vi "Script Add Constant VI.vi"(4 "Project Ref":refnum<vi>, 6 "App Ref":refnum<vi>, 7 "Constant VI Name":string="TESTING.vi", 8 "error in":errorcluster, 9 "Constant VI Args":refnum<vi>, 10 "Library Reference":refnum<vi>) -> (0 "error out":errorcluster)   [LabVIEW 2020, in "ConstantErrorsMaker.lvlib"]
uses:
  ConstantErrorsMaker.lvlib
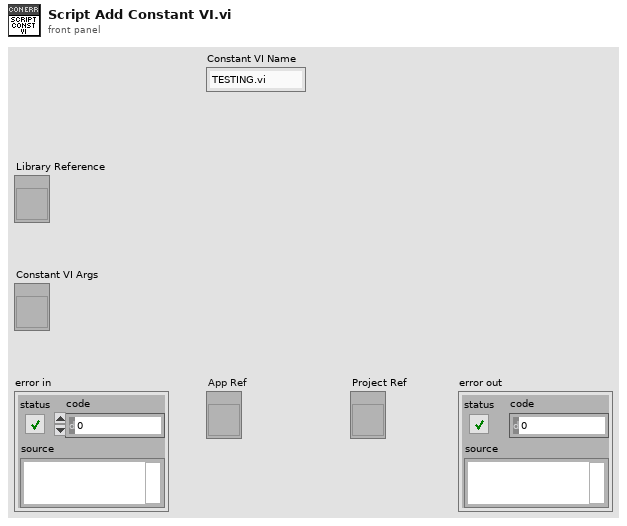
[diagram p1: front panel]
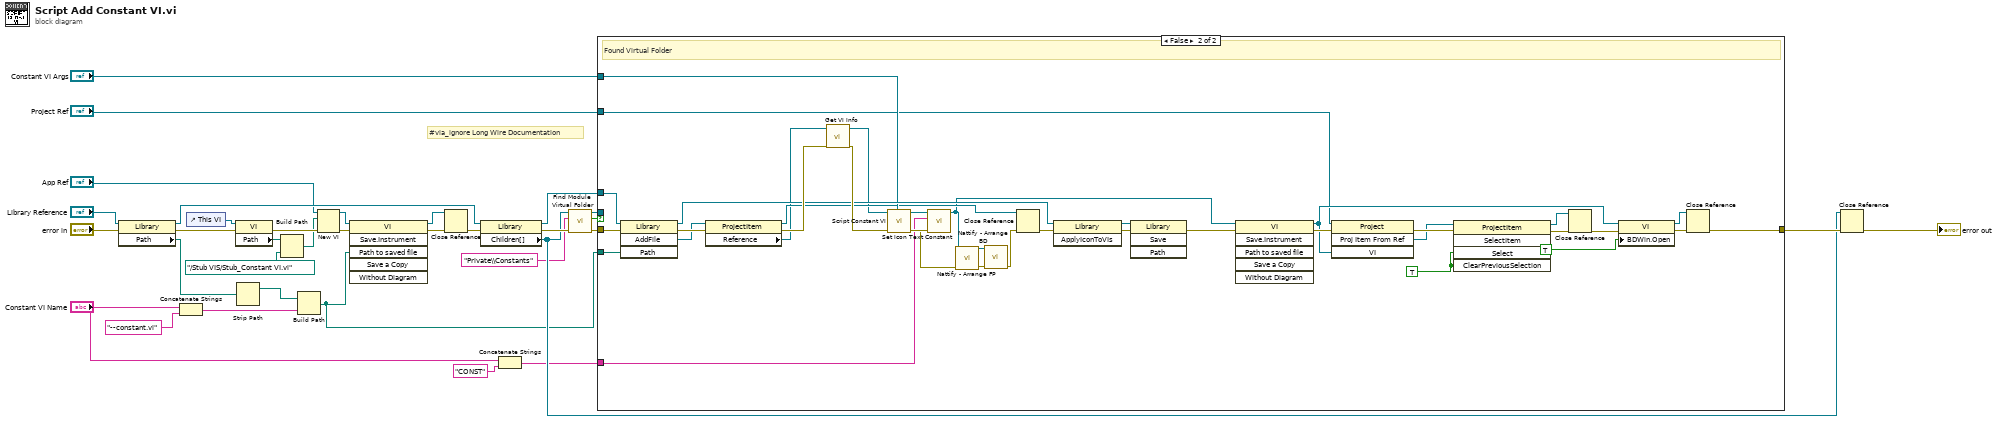
[diagram p0: block diagram]
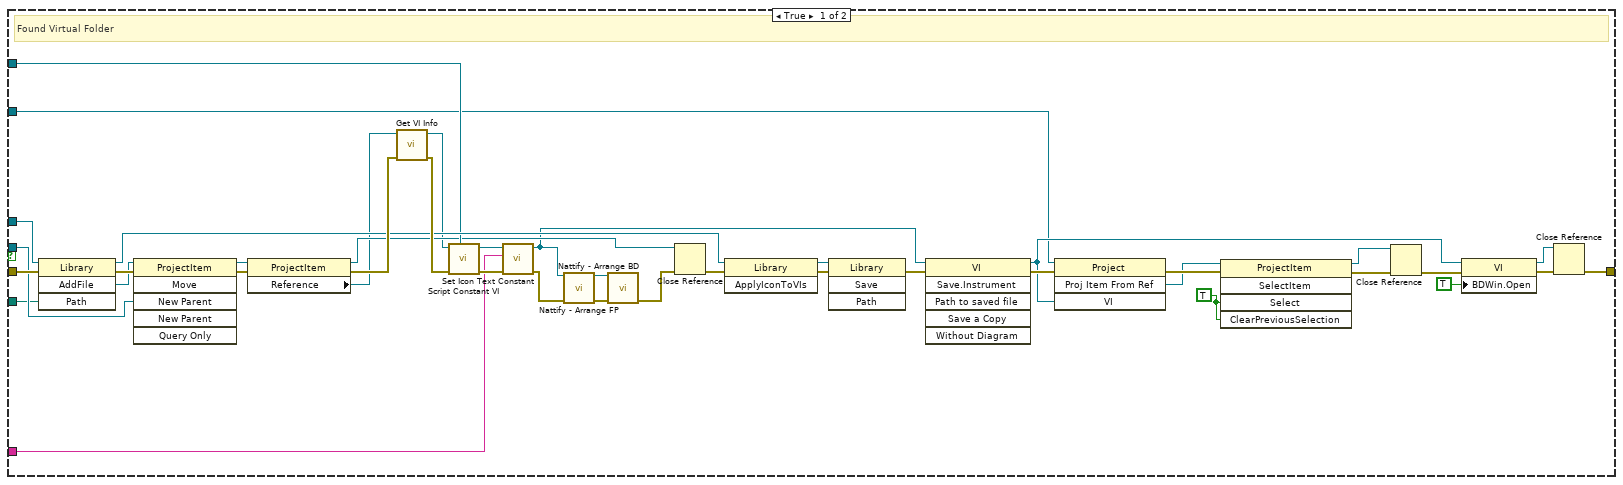
[diagram p2: hidden frame]
diagram:
  # "#via_ignore Long Wire Documentation"
  n1 = property class="Library"(reference="Library Reference", error in="error in") -> (reference out=w23:refnum<vi>, error out=w31:errorcluster, "Path"=w12:path)
  n2 = Concatenate Strings("Constant VI Name", "--constant.vi" ("input 1")) -> (w11:string)
  n3 = control-ref of="This VI"() -> (w10:refnum<vi>)
  n4 = property class="VI"(reference=w10, error in=w31) -> (error out=w25:errorcluster, "Path"=w9:path)  [unwired: 1 out]
  n5 = Strip Path(path=w12) -> (stripped path=w14:path)  [unwired: 1 out]
  n6 = Build Path(base path=w9, name or relative path=path "../Stub VIS/Stub_Constant VI.vi") -> (appended path=w8:path)
  n7 = Build Path(base path=w14, name or relative path=w11) -> (appended path=w13:path)
  n8 = New VI(8:w25, 10:w8, 11:"App Ref") -> (0:w28:errorcluster, 3:w16:refnum<vi>)  [unwired: 4 in]
  n9 = invoke class="VI" method="Save.Instrument"(reference=w16, error in=w28, "Path to saved file"=w13) -> (reference out=w6:refnum<vi>, error out=w26:errorcluster)  [unwired: 3 in, 4 out]
  n10 = Close Reference(reference=w6, error in (no error)=w26) -> (error out=w27:errorcluster)
  n11 = property class="Library"(reference=w23, error in=w27) -> (reference out=w24:refnum<vi>, error out=w33:errorcluster, "Children[]"=w20:refnum<vi>[])
  n12 = Concatenate Strings("Constant VI Name", "CONST" ("string")) -> (w2:string)
  n13 = call "Find Module Virtual Folder.vi"("error in"=w33, "Virtual Folder"="Private\\Constants", "Children"=w20) -> ("error out"=w32:errorcluster, "Found?"=w21:bool, "ProjectItem out"=w22:refnum<vi>)  [unwired: 6 in]
  n14 = case shown="False" w21 {
    tunnel: [w63 w101] -> w34
    tunnel: w24 -> [w56 w94]
    tunnel: w32 -> [w74 w111]
    tunnel: w22 -> [w54 _]
    tunnel: "Constant VI Args" -> [w50 w89]
    tunnel: w13 -> [w51 w90]
    tunnel: w2 -> [w42 w82]
    tunnel: "Project Ref" -> [w37 w78]
    frame True {
      w40 = TRUE ("Select")
      # "Found Virtual Folder"
      n15 = invoke class="Library" method="AddFile"(reference=w56, error in=w74, "Path"=w51) -> (reference out=w53:refnum<vi>, error out=w73:errorcluster, "AddFile"=w55:refnum<vi>)  [unwired: 1 in, 1 out]
      n16 = invoke class="ProjectItem" method="Move"(reference=w55, error in=w73, "New Parent"=w54) -> (reference out=w48:refnum<vi>, error out=w70:errorcluster)  [unwired: 3 in, 4 out]
      n17 = property class="ProjectItem"(reference=w48, error in=w70) -> (reference out=w47:refnum<vi>, error out=w58:errorcluster, "Reference"=w36:refnum<vi>)
      n18 = call "Get VI Info.vi"("error in"=w58, "VI in"=w36) -> ("error out"=w57:errorcluster, "VI out"=w35:refnum<vi>)  [unwired: 4 in, 4 out]
      n19 = call "Script Constant VI.vi"("Custom Argument Window"=w50, "error in"=w57, "VI Reference"=w35) -> ("error out"=w69:errorcluster, "VI reference"=w49:refnum<vi>)  [unwired: 7 in]
      n20 = call "Set Icon Text Constant.vi"("error in"=w69, "Text"=w42, "VI in"=w49) -> ("error out"=w67:errorcluster, "VI out"=w45:refnum<vi>)  [unwired: 7 in]
      n21 = call "Nattify - Arrange FP.vi"("VI in"=w45, "error in"=w67) -> ("VI out"=w46:refnum<vi>, "error out"=w68:errorcluster)  [unwired: 12 in]
      n22 = call "Nattify - Arrange BD.vi"("VI in"=w46, "error in"=w68) -> ("error out"=w65:errorcluster)  [unwired: 13 in]
      n23 = Close Reference(reference=w47, error in (no error)=w65) -> (error out=w71:errorcluster)
      n24 = invoke class="Library" method="ApplyIconToVIs"(reference=w53, error in=w71) -> (reference out=w52:refnum<vi>, error out=w72:errorcluster)  [unwired: 1 in, 1 out]
      n25 = invoke class="Library" method="Save"(reference=w52, error in=w72) -> (error out=w64:errorcluster)  [unwired: 2 in, 3 out]
      n26 = invoke class="VI" method="Save.Instrument"(reference=w45, error in=w64) -> (reference out=w39:refnum<vi>, error out=w61:errorcluster)  [unwired: 4 in, 4 out]
      n27 = invoke class="Project" method="Proj Item From Ref"(reference=w37, error in=w61, "VI"=w39) -> (error out=w62:errorcluster, "ProjItemFromRef"=w41:refnum<vi>)  [unwired: 1 in, 2 out]
      n28 = invoke class="ProjectItem" method="SelectItem"(reference=w41, error in=w62, "Select"=w40, "ClearPreviousSelection"=w40) -> (reference out=w38:refnum<vi>, error out=w60:errorcluster)  [unwired: 1 in, 3 out]
      n29 = Close Reference(reference=w38, error in (no error)=w60) -> (error out=w59:errorcluster)
      n30 = property class="VI"(reference=w39, error in=w59, "BDWin.Open"=TRUE ("Block Diagram Window:Open")) -> (reference out=w43:refnum<vi>, error out=w66:errorcluster)
      n31 = Close Reference(reference=w43, error in (no error)=w66) -> (error out=w63:errorcluster)
    }
    frame False {
      w80 = TRUE ("Select")
      # "Found Virtual Folder"
      n32 = invoke class="Library" method="AddFile"(reference=w94, error in=w111, "Path"=w90) -> (reference out=w92:refnum<vi>, error out=w100:errorcluster, "AddFile"=w93:refnum<vi>)  [unwired: 1 in, 1 out]
      n33 = property class="ProjectItem"(reference=w93, error in=w100) -> (reference out=w87:refnum<vi>, error out=w107:errorcluster, "Reference"=w76:refnum<vi>)
      n34 = call "Get VI Info.vi"("error in"=w107, "VI in"=w76) -> ("error out"=w95:errorcluster, "VI out"=w75:refnum<vi>)  [unwired: 4 in, 4 out]
      n35 = call "Script Constant VI.vi"("Custom Argument Window"=w89, "error in"=w95, "VI Reference"=w75) -> ("error out"=w108:errorcluster, "VI reference"=w88:refnum<vi>)  [unwired: 7 in]
      n36 = call "Set Icon Text Constant.vi"("error in"=w108, "Text"=w82, "VI in"=w88) -> ("error out"=w105:errorcluster, "VI out"=w85:refnum<vi>)  [unwired: 7 in]
      n37 = call "Nattify - Arrange FP.vi"("VI in"=w85, "error in"=w105) -> ("VI out"=w86:refnum<vi>, "error out"=w106:errorcluster)  [unwired: 12 in]
      n38 = call "Nattify - Arrange BD.vi"("VI in"=w86, "error in"=w106) -> ("error out"=w103:errorcluster)  [unwired: 13 in]
      n39 = Close Reference(reference=w87, error in (no error)=w103) -> (error out=w109:errorcluster)
      n40 = invoke class="Library" method="ApplyIconToVIs"(reference=w92, error in=w109) -> (reference out=w91:refnum<vi>, error out=w110:errorcluster)  [unwired: 1 in, 1 out]
      n41 = invoke class="Library" method="Save"(reference=w91, error in=w110) -> (error out=w102:errorcluster)  [unwired: 2 in, 3 out]
      n42 = invoke class="VI" method="Save.Instrument"(reference=w85, error in=w102) -> (reference out=w79:refnum<vi>, error out=w98:errorcluster)  [unwired: 4 in, 4 out]
      n43 = invoke class="Project" method="Proj Item From Ref"(reference=w78, error in=w98, "VI"=w79) -> (error out=w99:errorcluster, "ProjItemFromRef"=w81:refnum<vi>)  [unwired: 1 in, 2 out]
      n44 = invoke class="ProjectItem" method="SelectItem"(reference=w81, error in=w99, "Select"=w80, "ClearPreviousSelection"=w80) -> (reference out=w77:refnum<vi>, error out=w97:errorcluster)  [unwired: 1 in, 3 out]
      n45 = Close Reference(reference=w77, error in (no error)=w97) -> (error out=w96:errorcluster)
      n46 = property class="VI"(reference=w79, error in=w96, "BDWin.Open"=TRUE ("Block Diagram Window:Open")) -> (reference out=w83:refnum<vi>, error out=w104:errorcluster)
      n47 = Close Reference(reference=w83, error in (no error)=w104) -> (error out=w101:errorcluster)
    }
  }
  n48 = Close Reference(reference=w20, error in (no error)=w34) -> (error out=→"error out":errorcluster)
